vi "Find_Focus.vi"(8 "error in (no error)":errorcluster, 10 "Input_Z":dbl[](array[numeric])=[1.0, 2.0, 3.0, 4.0], 11 "Imput images":T1) -> (0 "error out":errorcluster, 3 "BestPosition":dbl)   [LabVIEW 2014]
doc: "This subVI is used to calculate the focus plane coordinate, calling a C++ dll."
uses:
  TypeDef/inputImages.ctl
  dll/focus_img.dll
  dll/focus_array.dll
panel:
  # "This subVI is used to calculate the focus plane coordinate, calling a C++ dll."
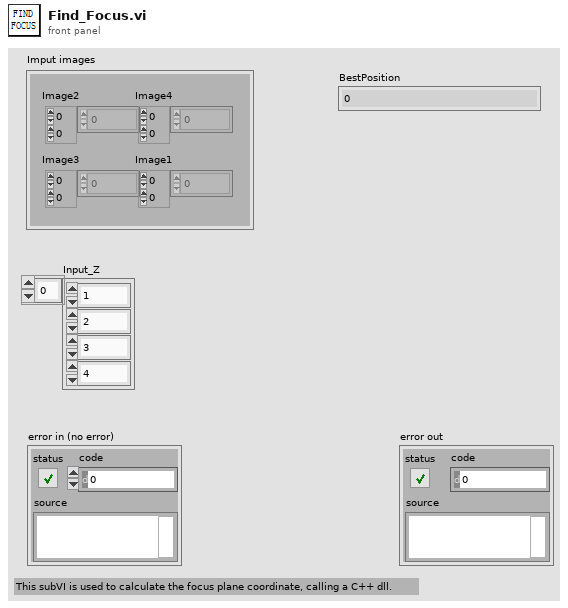
[diagram p1: front panel]
types:
  T1 = typedef "inputImages.ctl" = cluster{"Image2":u8[][], "Image3":u8[][], "Image4":u8[][], "Image1":u8[][]}
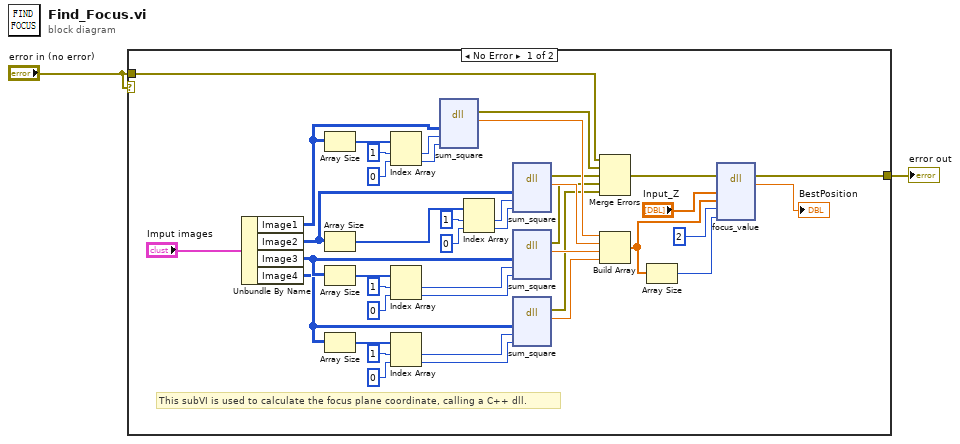
[diagram p0: block diagram]
diagram:
  n1 = case shown="No Error" "error in (no error)" {
    tunnel: [w4 w44] -> w2
    tunnel: "error in (no error)" -> [w3 w44]
    frame No Error {
      # "This subVI is used to calculate the focus plane coordinate, calling a C++ dll."
      n2 = Unbundle By Name("Imput images") -> ("Image1"=w15:u8[][], "Image2"=w14:u8[][], "Image3"=w13:u8[][], "Image4"=w12:u8[][])
      n3 = Array Size(array=w15) -> (size(s)=w41:i32[])
      n4 = Array Size(array=w14) -> (size(s)=w32:i32[])
      n5 = Array Size(array=w13) -> (size(s)=w31:i32[])
      n6 = Array Size(array=w12) -> (size(s)=w22:i32[])
      n7 = Index Array(array=w41, index #1=1 ("index"), index #2=0 ("index")) -> (element #1=w38:i32, element #2=w37:i32)
      n8 = Index Array(array=w31, index #1=1 ("index"), index #2=0 ("index")) -> (element #1=w28:i32, element #2=w27:i32)
      n9 = Index Array(array=w22, index #1=1 ("index"), index #2=0 ("index")) -> (element #1=w25:i32, element #2=w26:i32)
      n10 = dll-call lib="C:/Users/light/Desktop/Peng/Raman/dll/focus_img.dll" fn="sum_square" label="Sum_square"("pBuffer"=w15, "width"=w38, "height"=w37) -> (error out=w9:errorcluster, "return type"=w42:dbl)  [unwired: 6 in, 1 out]
      n11 = Index Array(array=w32, index #1=1 ("index"), index #2=0 ("index")) -> (element #1=w35:i32, element #2=w36:i32)
      n12 = dll-call lib="C:/Users/light/Desktop/Peng/Raman/dll/focus_img.dll" fn="sum_square"("pBuffer"=w14, "width"=w35, "height"=w36) -> (error out=w8:errorcluster, "return type"=w21:dbl)  [unwired: 6 in, 1 out]
      n13 = dll-call lib="C:/Users/light/Desktop/Peng/Raman/dll/focus_img.dll" fn="sum_square"("pBuffer"=w13, "width"=w28, "height"=w27) -> (error out=w7:errorcluster, "return type"=w20:dbl)  [unwired: 6 in, 1 out]
      n14 = dll-call lib="C:/Users/light/Desktop/Peng/Raman/dll/focus_img.dll" fn="sum_square"("pBuffer"=w12, "width"=w25, "height"=w26) -> (error out=w6:errorcluster, "return type"=w19:dbl)  [unwired: 6 in, 1 out]
      n15 = Merge Errors(w3, w9, w8, w7, w6) -> (w5:errorcluster)
      n16 = Build Array(w42, w21, w20, w19) -> (w11:dbl[])
      n17 = Array Size(array=w11) -> (size(s)=w10:i32)
      n18 = dll-call lib="C:/Users/light/Desktop/Peng/Raman/dll/focus_array.dll" fn="focus_value" label="Focus_value"(error in=w5, "x"="Input_Z", "y"=w11, "pow"=2, "total"=w10) -> (error out=w4:errorcluster, "return type"=→"BestPosition":dbl)  [unwired: 6 in, 1 out]
    }
    frame Error {
    }
  }
  "error out" <- w2
